vi "set_pixel_frequency.vi"(8 "error in (no error)":errorcluster, 10 "pixel dwell time":dbl[unit], 11 "FPGAWrapperMH120124RAPS_PXI7813R in":refnum<class "FPGAWrapperMH120124RAPS_PXI7813R.lvclass">) -> (0 "error out":errorcluster, 3 "FPGAWrapperMH120124RAPS_PXI7813R out":refnum<class "FPGAWrapperMH120124RAPS_PXI7813R.lvclass">)   [LabVIEW 2010, in "FPGAWrapperMH120124RAPS_PXI7813R.lvclass"]
uses:
  FPGAWrapperMH120124RAPS_PXI7813R.lvclass
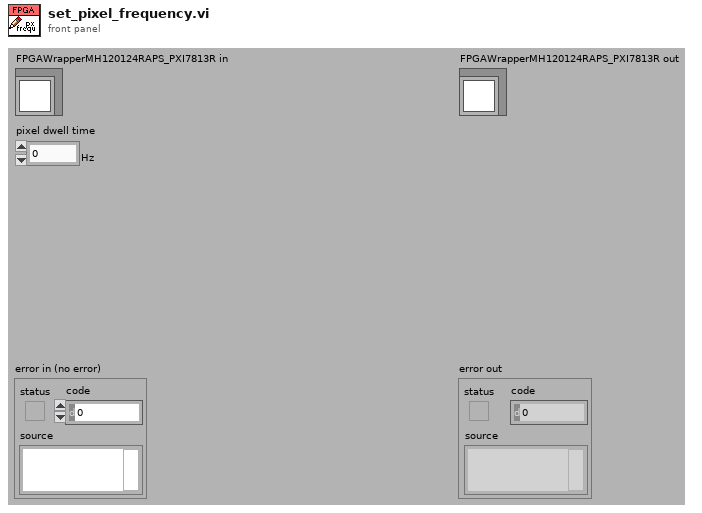
[diagram p1: front panel]
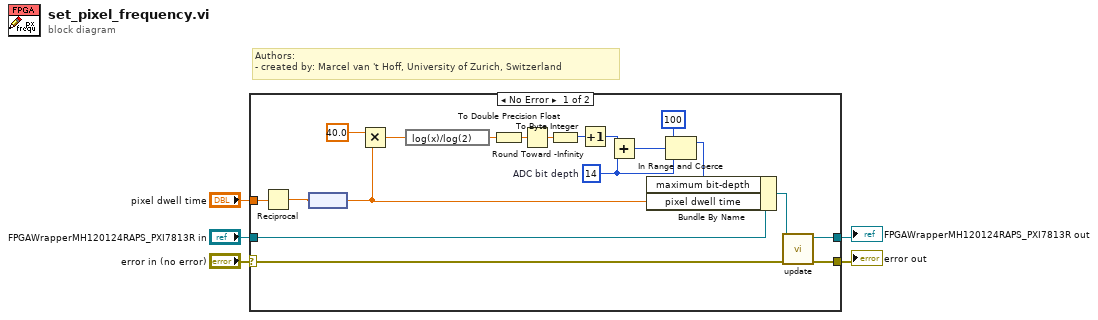
[diagram p0: block diagram]
diagram:
  # "Authors: \n- created by: Marcel van 't Hoff, University of Zurich, Switzerland"
  n1 = case shown="No Error" "error in (no error)" {
    selector: "error in (no error)" -> [w23 w25]
    tunnel: [w20 w25] -> w4
    tunnel: [w21 w26] -> w2
    tunnel: "FPGAWrapperMH120124RAPS_PXI7813R in" -> [w24 w26]
    tunnel: "pixel dwell time" -> [w7 _]
    frame No Error {
      w17 = i8 14  # ADC bit depth
      n2 = Reciprocal(x=w7) -> (1/x=w6:dbl[unit])
      n3 = node(w6) -> (w9:dbl)
      n4 = Multiply(x=40.0, y=w9) -> (x*y=w11:dbl)
      n5 = expression code="log(x)/log(2)"(w11) -> (w12:dbl)
      n6 = To Double Precision Float(number=w12) -> (double precision float=w14:dbl)
      n7 = Round Toward -Infinity(1:w14) -> (0:w13:dbl)
      n8 = To Byte Integer(number=w13) -> (8bit integer=w15:i8)
      n9 = Increment(x=w15) -> (x+1=w16:i8)
      n10 = Add(x=w16, y=w17) -> (x+y=w18:i8)
      n11 = In Range and Coerce(upper limit=i8 100, x=w18, lower limit=w17) -> (coerced(x)=w8:i8)  [unwired: 1 out]
      n12 = Bundle By Name(cluster=w24, "maximum bit-depth"=w8, "pixel dwell time"=w9) -> (w22:refnum<class "FPGAWrapperMH120124RAPS_PXI7813R.lvclass">)
      n13 = call-dynamic "update.vi"("error in (no error)"=w23, "FPGAWrapperMH120124RAPS_PXI7813R in"=w22) -> ("error out"=w20:errorcluster, "FPGAWrapperMH120124RAPS_PXI7813R out"=w21:refnum<class "FPGAWrapperMH120124RAPS_PXI7813R.lvclass">)  [unwired: 8 in]
    }
    frame Error {
    }
  }
  "error out" <- w4
  "FPGAWrapperMH120124RAPS_PXI7813R out" <- w2
